vi "ParamProg.vi"(8 "ErrorIn(No Error)":errorcluster caption="entrée d'erreur (pas d'erreur)", 11 "Interface.lvclass":refnum<class "Interface.lvclass">) -> (0 "sortie d'erreur":errorcluster, 2 "CheminOut":path, 3 "Interface.lvclass Out":refnum<class "Interface.lvclass">)   [LabVIEW 2010, in "Interface.lvclass"]
uses:
  Interface.lvclass
  Interface.lvclass/Interface.ctl
  SetInitPar.ctl
panel:
  in  "Startup":bool
  in  "Quit":bool
  in  "Save":bool
  in  "Chemin":path
  # "Chemin de sauvegarde"
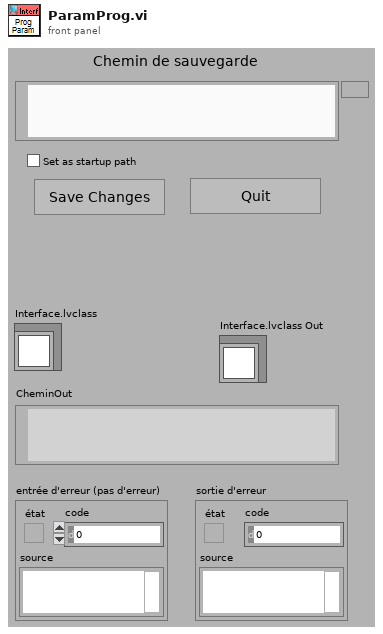
[diagram p1: front panel]
types:
  T1 = typedef "SetInitPar.ctl" = enum16{"All", "GraphConfig", "ScanFormats", "ScanPref", "LogPref", "BasePath", "Experiment"}
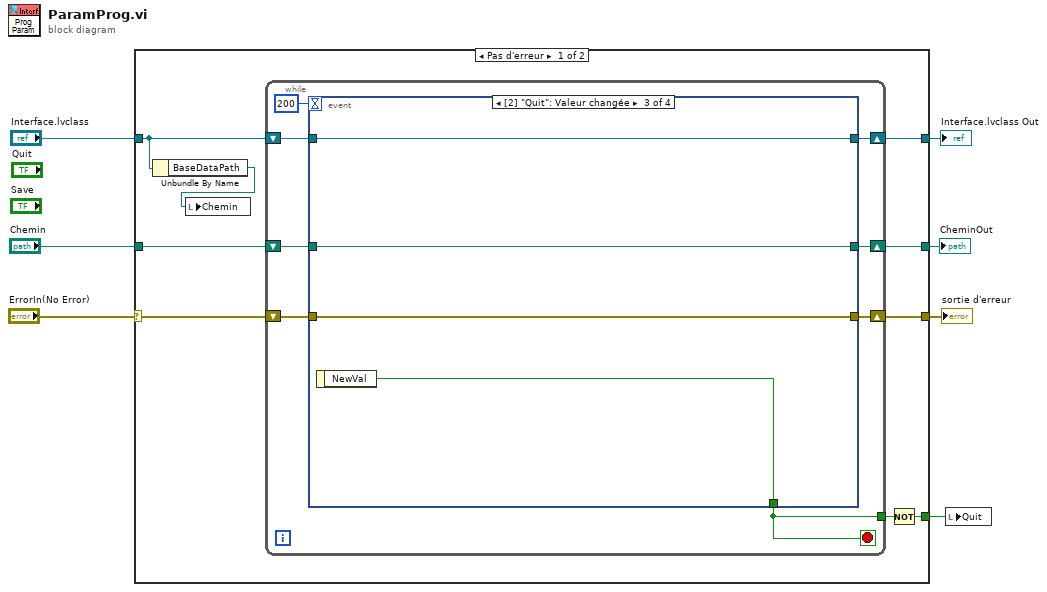
[diagram p0: block diagram]
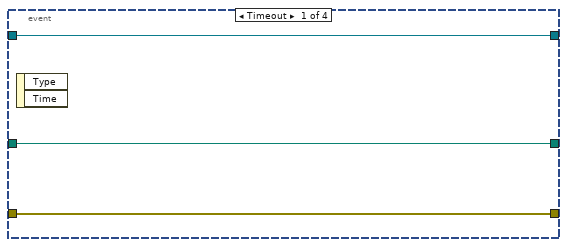
[diagram p2: hidden frame]
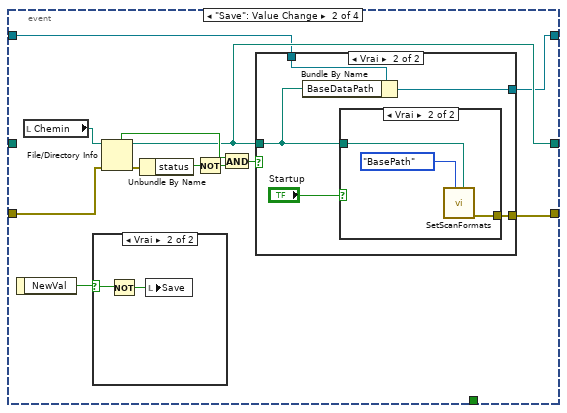
[diagram p3: hidden frame]
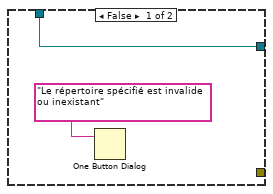
[diagram p4: hidden frame]
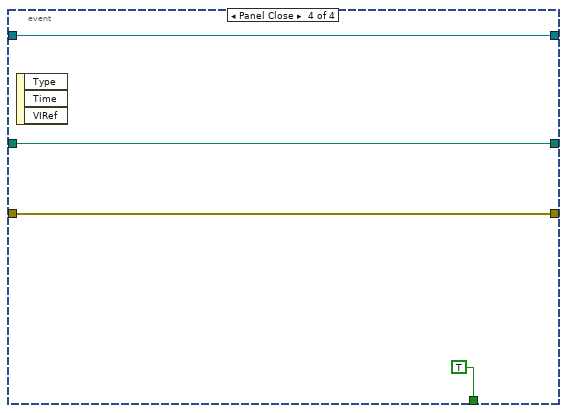
[diagram p7: hidden frame]
diagram:
  n1 = case shown="Pas d'erreur" "ErrorIn(No Error)" {
    selector: "ErrorIn(No Error)" -> [w16 w62]
    tunnel: [w14 w62] -> w6
    tunnel: "Chemin" -> [w15 w61]
    tunnel: [w13 w61] -> w5
    tunnel: [w11 _] -> w4
    tunnel: "Interface.lvclass" -> [w9 w60]
    tunnel: [w8 w60] -> w1
    frame No Error {
      n2 = Unbundle By Name(w9) -> ("BaseDataPath"=w10:path)
      n3 = local write "Chemin"(w10) -> ()
      n4 = while {
        shift-right: [w21] -> w14
        shift-left: w16 -> [w22]
        shift-right: [w23] -> w13
        shift-left: w15 -> [w24]
        tunnel: [w19] -> w12
        shift-right: [w17] -> w8
        shift-left: w9 -> [w18]
        stop <- w19 stop-if-true
        n5 = event shown="[2] \"Quit\": Valeur changée" {
          selector: _ -> [_ _ _ _]
          dyn-events: _ -> [_ _ _ _]
          timeout: 200 -> [_ _ _ _]
          tunnel: [_ _ w55 TRUE] -> w19
          tunnel: w24 -> [w27 _ w53 w57]
          tunnel: [w27 w30 w53 w57] -> w23
          tunnel: w22 -> [w26 w36 w54 w58]
          tunnel: [w26 w38 w54 w58] -> w21
          tunnel: w18 -> [w25 w29 w52 w56]
          tunnel: [w25 w28 w52 w56] -> w17
          event Timeout {
            n6 = event-data() -> ()  [unwired: 1 in, 2 out]
          }
          event "Save": Value Change {
            n7 = event-data() -> ("NewVal"=w39:bool)  [unwired: 1 in]
            n8 = local read "Chemin"() -> (w37:path)
            n9 = case shown="Vrai" w39 {
              selector: w39 -> [_ w51]
              frame False {
              }
              frame True {
                n10 = Not(x=w51) -> (.not. x?=w50:bool)
                n11 = local write "Save"(w50) -> ()
              }
            }
            n12 = File/Directory Info(path=w37, error in=w36) -> (path out=w30:path, directory=w31:bool, error out=w35:errorcluster)  [unwired: 4 out]
            n13 = Unbundle By Name(w35) -> ("status"=w33:bool)
            n14 = Not(x=w33) -> (.not. x?=w32:bool)
            n15 = And(x=w31, y=w32) -> (x .and. y?=w34:bool)
            n16 = case shown="Vrai" w34 {
              tunnel: [_ w46] -> w38
              tunnel: w30 -> [_ w43]
              tunnel: w29 -> [w40 w44]
              tunnel: [w40 w42] -> w28
              frame False {
                n17 = One Button Dialog(message="Le répertoire spécifié est invalide ou inexistant") -> ()  [unwired: 1 in, 1 out]
              }
              frame True {
                n18 = Bundle By Name(cluster=w44, "BaseDataPath"=w43) -> (w42:refnum<class "Interface.lvclass">)
                n19 = case shown="Vrai" "Startup" {
                  tunnel: [_ w49] -> w46
                  tunnel: w43 -> [_ w48]
                  frame False {
                  }
                  frame True {
                    n20 = call "SetScanFormats.vi"("Répertoire initial"=w48, "Énum"=SetInitPar."BasePath") -> ("sortie d'erreur"=w49:errorcluster)  [unwired: 9 in]
                  }
                }
              }
            }
          }
          event "Quit": Value Change {
            n21 = event-data() -> ("NewVal"=w55:bool)  [unwired: 1 in]
          }
          event Panel Close {
            n22 = event-data() -> ()  [unwired: 1 in, 3 out]
          }
        }
      }
      n23 = Not(x=w12) -> (.not. x?=w11:bool)
    }
    frame Error {
    }
  }
  "sortie d'erreur" <- w6
  "CheminOut" <- w5
  "Interface.lvclass Out" <- w1
  n24 = local write "Quit"(w4) -> ()
